vi "envio datos a uc.vi"(4 "ON  /  OFF":bool, 5 "Sentido de Giro 3":bool, 6 "VELOCIDAD (PWM 3- Duty Cicle)":dbl, 7 "Sentido de Giro 2":bool, 8 "VELOCIDAD (PWM 2 - Duty Cicle)":dbl, 9 "Sentido de Giro 1":bool, 10 "VELOCIDAD (PWM 1 - Duty Cicle)":dbl) -> (0 "Velocidad 3":dbl, 1 "Velocidad 2":dbl, 2 "Velocidad 1":dbl, 3 "String":string)   [LabVIEW 2018]
uses:
  <vilib>/express/express arith-compare/Formula/XNode/ExpressFormulaBlockNode.xnode
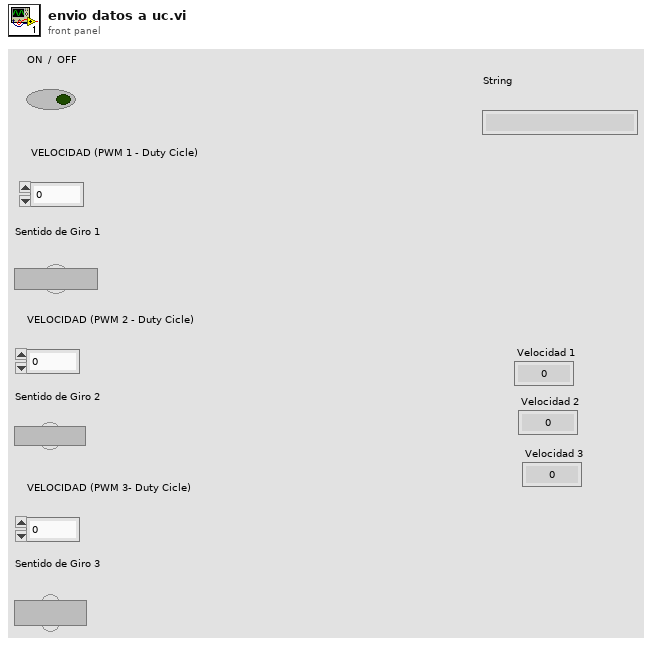
[diagram p1: front panel]
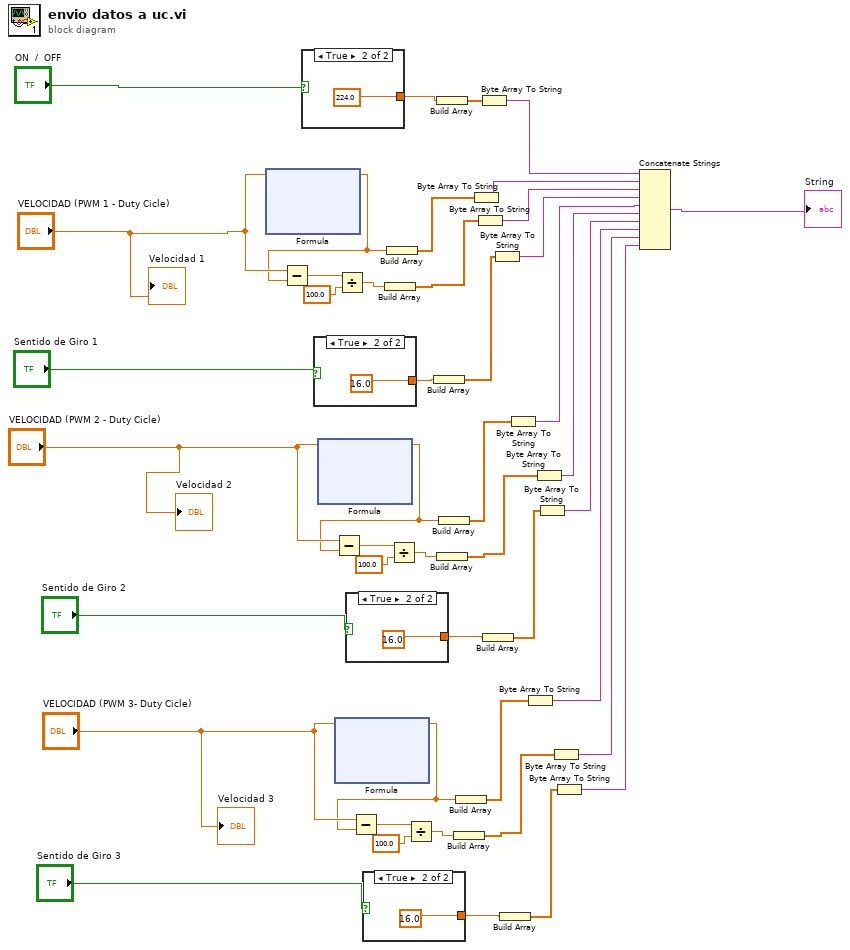
[diagram p0: block diagram]
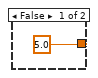
[diagram p2: hidden frame]
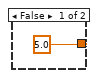
[diagram p3: hidden frame]
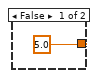
[diagram p4: hidden frame]
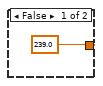
[diagram p5: hidden frame]
diagram:
  n1 = xnode "Formula"("X1"="VELOCIDAD (PWM 1 - Duty Cicle)") -> ("Result"=w2:dbl)  [unwired: 1 in, 1 out]
  n2 = Subtract(x="VELOCIDAD (PWM 1 - Duty Cicle)", y=w2) -> (x-y=w4:dbl)
  n3 = case shown="True" "ON  /  OFF" {
    tunnel: [239.0 ("element") 224.0 ("element")] -> w11
    frame False {
    }
    frame True {
    }
  }
  n4 = case shown="True" "Sentido de Giro 1" {
    tunnel: [5.0 ("element") 16.0 ("element")] -> w29
    frame False {
    }
    frame True {
    }
  }
  n5 = xnode "Formula"("X1"="VELOCIDAD (PWM 2 - Duty Cicle)") -> ("Result"=w18:dbl)  [unwired: 1 in, 1 out]
  n6 = Subtract(x="VELOCIDAD (PWM 2 - Duty Cicle)", y=w18) -> (x-y=w20:dbl)
  n7 = xnode "Formula"("X1"="VELOCIDAD (PWM 3- Duty Cicle)") -> ("Result"=w33:dbl)  [unwired: 1 in, 1 out]
  n8 = Divide(x=w4, y=100.0) -> (x/y=w1:dbl)
  n9 = case shown="True" "Sentido de Giro 2" {
    tunnel: [5.0 ("element") 16.0 ("element")] -> w24
    frame False {
    }
    frame True {
    }
  }
  n10 = Subtract(x="VELOCIDAD (PWM 3- Duty Cicle)", y=w33) -> (x-y=w35:dbl)
  n11 = case shown="True" "Sentido de Giro 3" {
    tunnel: [5.0 ("element") 16.0 ("element")] -> w39
    frame False {
    }
    frame True {
    }
  }
  n12 = Build Array(w1) -> (w6:dbl[])
  n13 = Build Array(w2) -> (w5:dbl[])
  n14 = Divide(x=w20, y=100.0) -> (x/y=w17:dbl)
  n15 = Divide(x=w35, y=100.0) -> (x/y=w32:dbl)
  n16 = Build Array(w29) -> (w28:dbl[])
  n17 = Build Array(w11) -> (w7:dbl[])
  n18 = Build Array(w17) -> (w22:dbl[])
  n19 = Build Array(w18) -> (w21:dbl[])
  n20 = Build Array(w32) -> (w37:dbl[])
  n21 = Build Array(w33) -> (w36:dbl[])
  n22 = Byte Array To String(unsigned byte array=w5) -> (string=w12:string)
  n23 = Byte Array To String(unsigned byte array=w6) -> (string=w13:string)
  n24 = Byte Array To String(unsigned byte array=w7) -> (string=w9:string)
  n25 = Build Array(w24) -> (w23:dbl[])
  n26 = Byte Array To String(unsigned byte array=w28) -> (string=w15:string)
  n27 = Build Array(w39) -> (w38:dbl[])
  n28 = Byte Array To String(unsigned byte array=w21) -> (string=w25:string)
  n29 = Byte Array To String(unsigned byte array=w36) -> (string=w42:string)
  n30 = Byte Array To String(unsigned byte array=w22) -> (string=w26:string)
  n31 = Byte Array To String(unsigned byte array=w23) -> (string=w27:string)
  n32 = Byte Array To String(unsigned byte array=w37) -> (string=w43:string)
  n33 = Byte Array To String(unsigned byte array=w38) -> (string=w44:string)
  n34 = Concatenate Strings(w9, w12, w13, w15, w25, w26, w27, w42, w43, w44) -> (→"String":string)
  "Velocidad 1" <- "VELOCIDAD (PWM 1 - Duty Cicle)"
  "Velocidad 2" <- "VELOCIDAD (PWM 2 - Duty Cicle)"
  "Velocidad 3" <- "VELOCIDAD (PWM 3- Duty Cicle)"
